vi "Boolean to Yes or No.vi"(4 "Boolean":bool) -> (0 "lowercase":string, 1 "UPPERCASE":string, 2 "Capitalized":string)   [LabVIEW 2020, in "Utilities.lvlib"]
doc: "Converts a boolean to either \"Yes\" or \"No\". The string is returned capitalized, in all uppercase, and in all lowercase."
uses:
  Utilities.lvlib
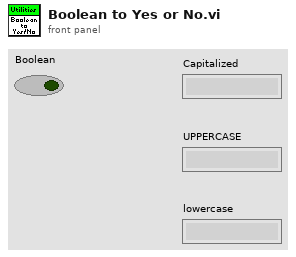
[diagram p1: front panel]
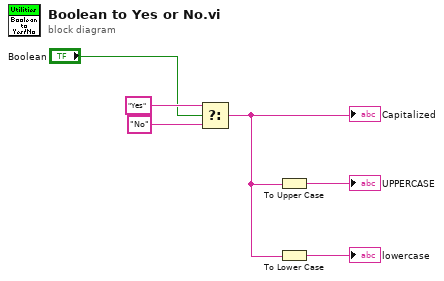
[diagram p0: block diagram]
diagram:
  n1 = Select(t="Yes", s="Boolean", f="No") -> (s? t:f=w2:string)
  "Capitalized" <- w2
  n2 = To Upper Case(1:w2) -> (0:→"UPPERCASE":string)
  n3 = To Lower Case(string=w2) -> (all lower case string=→"lowercase":string)
